vi "SA Initialize - NF.vi"(8 "error in":errorcluster, 9 "Test Configuration":T1={"Y-Factor Mode"=0, "Measurement Bandwidth (Hz)"=4000000.0, "Measurement Interval (s)"=0.1, "NF Cal Setup ID"="SNS_PS_6dB_ENR15_26.5GHz_VI", "NF DUT Type"=0, "Frequency List (Hz)"=[4000000000.0, 5000000000.0, 6000000000.0, 7000000000.0, 8000000000.0, 9000000000.0, 10000000000.0, 11000000000.0, 12000000000.0, 13000000000.0, 14000000000.0, 15000000000.0, 16000000000.0, 17000000000.0, 18000000000.0, 19000000000.0, 20000000000.0], "Averaging"={"Enabled"=0, "Count"=10}, "Noise Source"={"Noise Source Type"=1, "Noise Source RFSG Port"="", "Cold Temperature (K)"=302.8, "Off Temperature (K)"=297.0, "ENR Freq (Hz)"=[6500000000.0], "ENR (dB)"=[15.0]}} {"Frequency List (Hz)" format="%.3p"; "NF DUT Type" items=["Amplifier", "Downconverter", "Upconverter"]; "Y-Factor Mode" items=["Measure", "Calibrate"]; "Noise Source"."Noise Source Type" items=["External Noise Source", "RF Signal Generator"]; "Noise Source"."ENR (dB)" format="%.2g"; "Noise Source"."ENR Freq (Hz)" format="%.3p"; "Noise Source"."Off Temperature (K)" format="%.2f"; "Noise Source"."Cold Temperature (K)" format="%.2f"; "Averaging"."Enabled" items=["False", "True"]; "Measurement Interval (s)" format="%.2p"; "Measurement Bandwidth (Hz)" format="%.3p"}, 10 "RFmx Settings":T2={"RFmx Name"="", "RFmx Port"="", "Reference Level"={"DUT Max Gain (dB)"=0.0, "DUT Max Noise Figure (dB)"=0.0, "Mode"=enum."Manual", "Reference Level (dBm)"=0.0}, "Preamp Enabled"=0, "Attenuation"={"Mode"=enum."Constant Attenuation", "Constant Attenuation"={"RFmx External Attenuation (dB)"=11.2}, "s2p File"={"RFmx S-Parameters Orientation"=24000, "RFmx Attenuation s2p File"=path ""}}, "ENS Source"={"SMU Name"="", "SMU Channel"=""}} {"Attenuation"."s2p File"."RFmx S-Parameters Orientation" items=["Port1 Towards DUT"=24000, "Port2 Towards DUT"=24001]; "Attenuation"."Constant Attenuation"."RFmx External Attenuation (dB)" format="%.2f"; "Preamp Enabled" items=["Disabled"=0, "Enabled"=1, "Automatic"=3]}) -> (0 "error out":errorcluster, 3 "RFmx Session out":refnum<k21>)   [LabVIEW 2023]
uses:
  Controls/RFmx Config - NF.ctl
  Controls/Test Config - NF.ctl
  FPT Shared VIs/De-embedding/RFmx Config.ctl
  <vilib>/RFmx/SpecAn/mx/RFmxSpecAn.llb/RFmxSpecAn Select Measurement (Single).vi
  <resource>/objmgr/RFmxSpecAn.rc
  <resource>/objmgr/RFmxInstr.rc
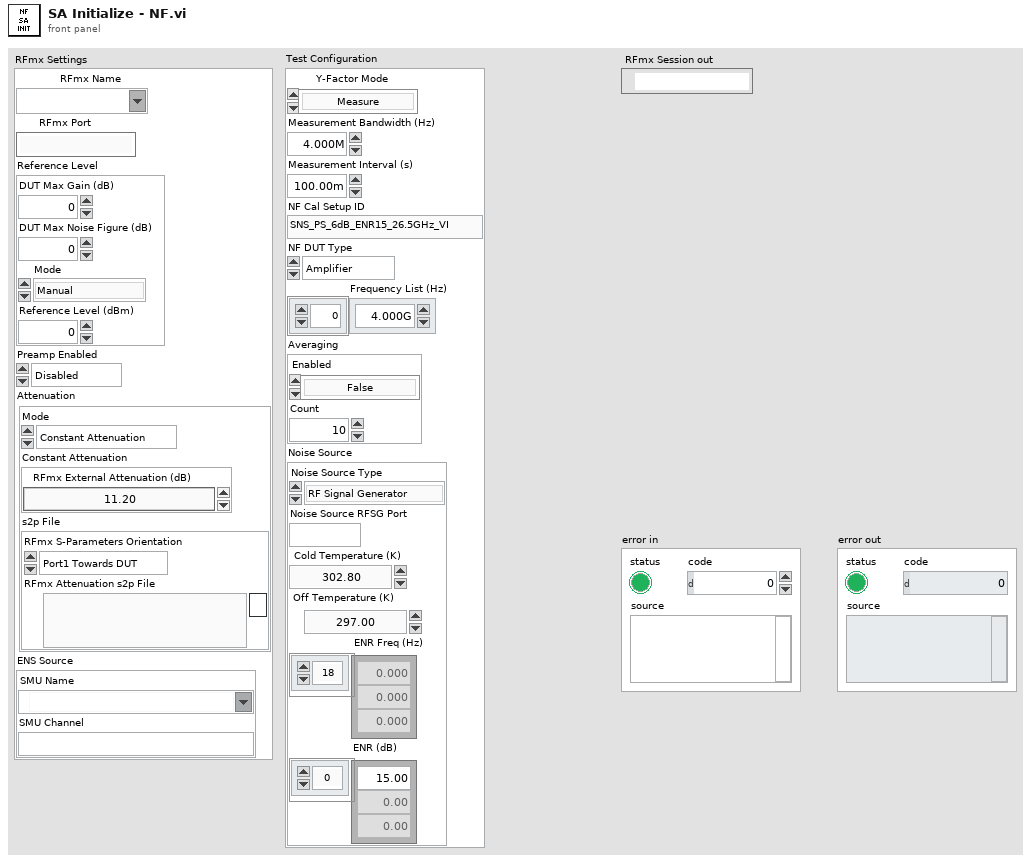
[diagram p1: front panel]
types:
  T1 = typedef "Test Config - NF.ctl" = cluster{"Y-Factor Mode":i32, "Measurement Bandwidth (Hz)":dbl, "Measurement Interval (s)":dbl, "NF Cal Setup ID":string, "NF DUT Type":i32, "Frequency List (Hz)":dbl[], "Averaging":cluster{"Enabled":i32, "Count":i32}, "Noise Source":cluster{"Noise Source Type":i32, "Noise Source RFSG Port":string, "Cold Temperature (K)":dbl, "Off Temperature (K)":dbl, "ENR Freq (Hz)":dbl[], "ENR (dB)":dbl[]}}
  T2 = typedef "RFmx Config - NF.ctl" = cluster{"RFmx Name":refnum<k15>, "RFmx Port":string, "Reference Level":cluster{"DUT Max Gain (dB)":dbl, "DUT Max Noise Figure (dB)":dbl, "Mode":enum32{"Manual", "Recommend"}, "Reference Level (dBm)":dbl}, "Preamp Enabled":i32, "Attenuation":cluster{"Mode":enum32{"<None>", "Constant Attenuation", "s2p File"}, "Constant Attenuation":cluster{"RFmx External Attenuation (dB)":dbl}, "s2p File":cluster{"RFmx S-Parameters Orientation":i32, "RFmx Attenuation s2p File":path}}, "ENS Source":cluster{"SMU Name":refnum<k15>, "SMU Channel":string}}
  T3 = typedef "RFmx Config.ctl" = cluster{"RFmx Name":refnum<k15>, "RFmx Port":string, "Attenuation":cluster{"Mode":enum32{"<None>", "Constant Attenuation", "s2p File"}, "Constant Attenuation":cluster{"RFmx External Attenuation (dB)":dbl}, "s2p File":cluster{"RFmx S-Parameters Orientation":i32, "RFmx Attenuation s2p Path Name":string, "RFmx Attenuation s2p File":path}}}
  T4 = enum16{"ACP", "CCDF", "CHP", "FCnt", "Harmonics", "OBW", "SEM", "Spectrum", "Spur", "TXP", "AMPM", "DPD", "IQ", "IM", "NF", "PhaseNoise", "PAVT", "IDPD"}
  T5 = enum32{"<None>", "Constant Attenuation", "s2p File"}
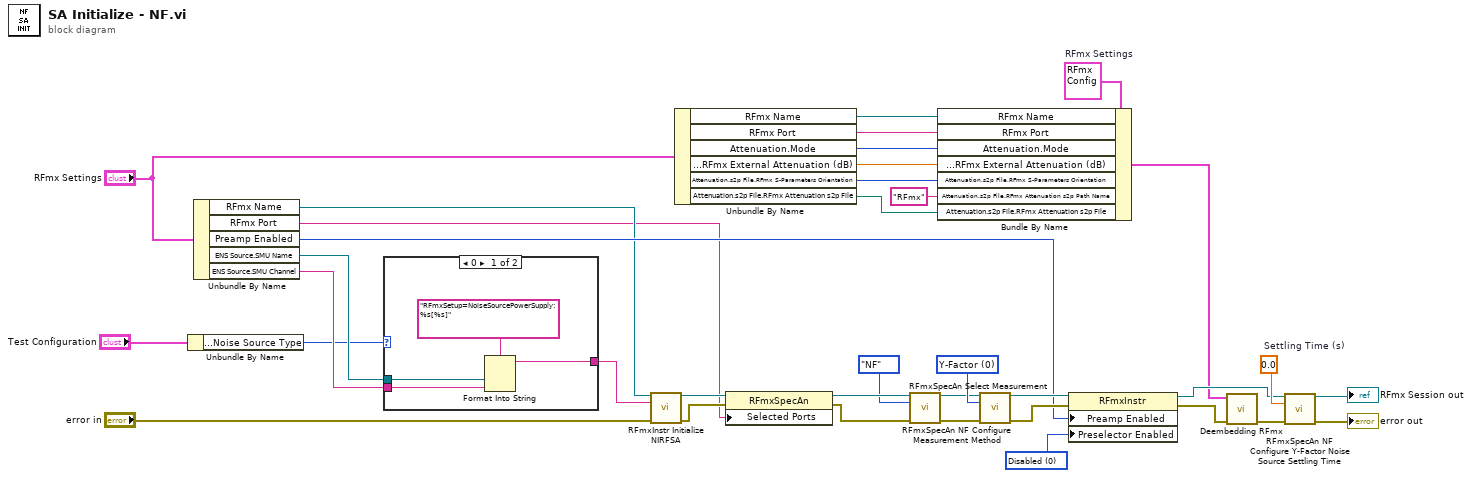
[diagram p0: block diagram]
diagram:
  w15 = T3 {"RFmx Name"="5842_0", "RFmx Port"="", "Attenuation"={"Mode"=enum."Constant Attenuation", "Constant Attenuation"={"RFmx External Attenuation (dB)"=1.2}, "s2p File"={"RFmx S-Parameters Orientation"=24000, "RFmx Attenuation s2p Path Name"="", "RFmx Attenuation s2p File"=path ""}}}  # RFmx Settings
  w23 = 0.0  # Settling Time (s)
  w34 = 0 items=["Disabled", "Enabled"] ("Preselector Enabled")
  w29 = 0 items=["Y-Factor", "Cold Source"] ("Measurement Method")
  n1 = Unbundle By Name("Test Configuration") -> ("Noise Source.Noise Source Type"=w1:i32)
  n2 = Unbundle By Name("RFmx Settings") -> ("RFmx Name"=w17:refnum<k15>, "RFmx Port"=w16:string, "Preamp Enabled"=w24:i32, "ENS Source.SMU Name"=w4:refnum<k15>, "ENS Source.SMU Channel"=w3:string)
  n3 = case shown="0" w1 {
    tunnel: [w39 _] -> w5
    tunnel: w4 -> [w38 _]
    tunnel: w3 -> [w37 _]
    frame 0 {
      n4 = Format Into String(format string="RFmxSetup=NoiseSourcePowerSupply:%s[%s]", w38, w37) -> (resulting string=w39:string)  [unwired: 2 in, 1 out]
    }
    frame 1, Default {
    }
  }
  n5 = call <vilib>:"RFmxInstr Initialize NIRFSA.vi"("Resource Name"=w17, "Option String"=w5, "error in (no error)"="error in") -> ("Instrument Handle Out"=w25:refnum<k21>, "error out"=w26:errorcluster)  [unwired: 10 in, 1 out]
  n6 = Unbundle By Name("RFmx Settings") -> ("RFmx Name"=w13:refnum<k15>, "RFmx Port"=w12:string, "Attenuation.Mode"=w8:T5, "Attenuation.Constant Attenuation.RFmx External Attenuation (dB)"=w11:dbl, "Attenuation.s2p File.RFmx S-Parameters Orientation"=w10:i32, "Attenuation.s2p File.RFmx Attenuation s2p File"=w9:path)
  n7 = property class="RFmxSpecAn"(reference=w25, error in=w26, "Selected Ports"=w16) -> (reference out=w32:refnum<k21>, error out=w30:errorcluster)
  n8 = call-poly <vilib>:"RFmxSpecAn Select Measurement.vi"("Instrument Handle In"=w32, "Measurement"=T4."NF", "error in (no error)"=w30) -> ("Instrument Handle Out"=w27:refnum<k21>, "error out"=w28:errorcluster)  [unwired: 11 in]
  n9 = Bundle By Name(cluster=w15, "RFmx Name"=w13, "RFmx Port"=w12, "Attenuation.Mode"=w8, "Attenuation.Constant Attenuation.RFmx External Attenuation (dB)"=w11, "Attenuation.s2p File.RFmx S-Parameters Orientation"=w10, "Attenuation.s2p File.RFmx Attenuation s2p Path Name"="RFmx", "Attenuation.s2p File.RFmx Attenuation s2p File"=w9) -> (w7:T3)
  n10 = call <vilib>:"RFmxSpecAn NF Configure Measurement Method.vi"("Instrument Handle In"=w27, "Measurement Method"=w29, "error in (no error)"=w28) -> ("Instrument Handle Out"=w35:refnum<k21>, "error out"=w36:errorcluster)  [unwired: 11 in]
  n11 = property class="RFmxInstr"(reference=w35, error in=w36, "Preamp Enabled"=w24, "Preselector Enabled"=w34) -> (reference out=w18:refnum<k21>, error out=w19:errorcluster)
  n12 = call "Deembedding RFmx.vi"("error in"=w19, "RFmx Settings"=w7) -> ("error out"=w20:errorcluster)  [unwired: 8 in, 1 out]
  n13 = call <vilib>:"RFmxSpecAn NF Configure Y-Factor Noise Source Settling Time.vi"("Instrument Handle In"=w18, "Settling Time (s)"=w23, "error in (no error)"=w20) -> ("Instrument Handle Out"=→"RFmx Session out":refnum<k21>, "error out"=→"error out":errorcluster)  [unwired: 11 in]
